vi "Control-IncrementSigma.vi"(0 "Señal de Control IN":dbl[](array[numeric]), 5 "Sound Parameters":cluster{"# samples":u32, "tiempos (ms)":dbl}, 7 "Parametros Actuales IN":T1, 9 "detla Parametros":T1, 11 "Parametros Maximos":T1) -> (4 "Out":dbl[](array[numeric]), 6 "Tope?":bool, 8 "Parametros Actuales OUT":T1)   [LabVIEW 2010]
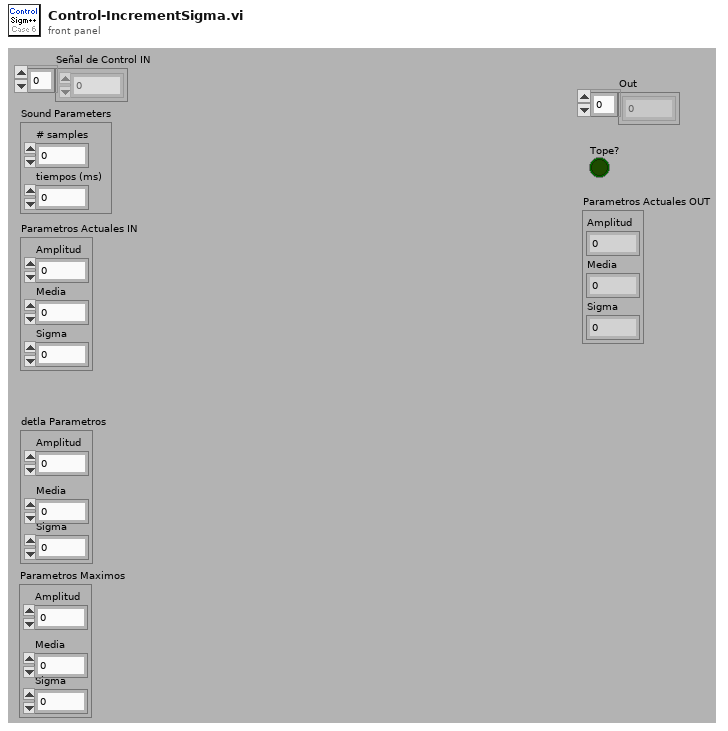
[diagram p1: front panel]
types:
  T1 = cluster{"Amplitud":dbl, "Media":dbl, "Sigma":dbl}
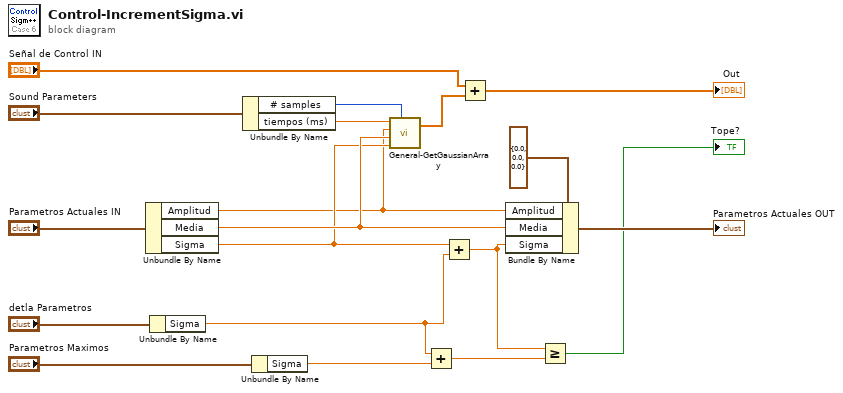
[diagram p0: block diagram]
diagram:
  n1 = Unbundle By Name("Parametros Actuales IN") -> ("Amplitud"=w4:dbl, "Media"=w7:dbl, "Sigma"=w5:dbl)
  n2 = Unbundle By Name("detla Parametros") -> ("Sigma"=w2:dbl)
  n3 = Unbundle By Name("Sound Parameters") -> ("# samples"=w12:u32, "tiempos (ms)"=w11:dbl)
  n4 = Unbundle By Name("Parametros Maximos") -> ("Sigma"=w3:dbl)
  n5 = call "General-GetGaussianArray.vi"("tiempo (ms)"=w11, "Amplitud"=w4, "t0 (ms)"=w7, "Sigma (ms)"=w5, "#samples"=w12) -> ("Y out"=w18:dbl[])  [unwired: 1 out]
  n6 = Add(x=w2, y=w3) -> (x+y=w1:dbl)
  n7 = Add(x=w5, y=w2) -> (x+y=w6:dbl)
  n8 = Add(x="Señal de Control IN", y=w18) -> (x+y=→"Out":dbl[])
  n9 = Bundle By Name(cluster=T1 {"Amplitud"=0.0, "Media"=0.0, "Sigma"=0.0} ("input cluster"), "Amplitud"=w4, "Media"=w7, "Sigma"=w6) -> (→"Parametros Actuales OUT":T1)
  n10 = Greater Or Equal?(x=w6, y=w1) -> (x >= y?=→"Tope?":bool)
